vi "Read scan period (uSec).vi"(8 "error in":errorcluster, 11 "timing source in":refnum<class "scan engine timing source.lvclass">) -> (0 "error out":errorcluster, 2 "scan period (uSec)":u32=10000, 3 "timing source out":refnum<class "scan engine timing source.lvclass">)   [LabVIEW 2013, in "scan engine timing source.lvclass"]
doc: "Reads the scan period of the scan engine source <b>as configured in the class, not in the system at the current moment</b>"
uses:
  scan engine timing source.lvclass
  scan engine timing source.lvclass/scan engine timing source.ctl
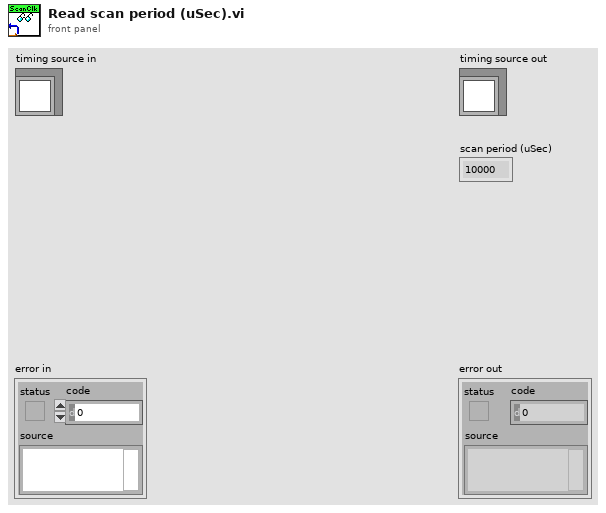
[diagram p1: front panel]
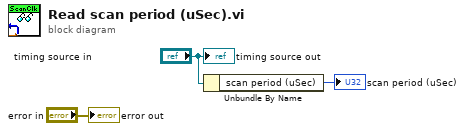
[diagram p0: block diagram]
diagram:
  n1 = Unbundle By Name("timing source in") -> ("scan period (uSec)"=→"scan period (uSec)":u32)
  "error out" <- "error in"
  "timing source out" <- "timing source in"
